vi "Initialize Attributes (public).vi"(8 "error in (no error)":errorcluster, 10 "Attribute Data":variant, 11 "CS++Base in":refnum<class "CS++Base.lvclass">) -> (0 "error out":errorcluster, 2 "Found?":bool, 3 "CS++Base out":refnum<class "CS++Base.lvclass">)   [LabVIEW 2015, in "CS++BaseClasses.lvlib" / "CS++Base.lvclass"]
doc: "Initialize object attribute.\n\nUnique resources should be allocated elsewhere!"
uses:
  CS++Base.lvclass
  CS++Base.lvclass/CS++Base.ctl
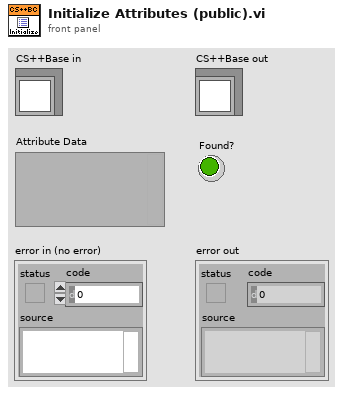
[diagram p1: front panel]
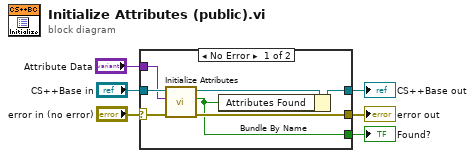
[diagram p0: block diagram]
diagram:
  n1 = case shown="No Error" "error in (no error)" {
    selector: "error in (no error)" -> [w12 w15]
    tunnel: [w11 w15] -> w5
    tunnel: [w8 w14] -> w3
    tunnel: "CS++Base in" -> [w13 w14]
    tunnel: "Attribute Data" -> [w10 _]
    tunnel: [w7 _] -> w1
    frame No Error {
      n2 = call-dynamic "Initialize Attributes.vi"("error in (no error)"=w12, "Attribute Data"=w10, "CS++Base in"=w13) -> ("error out"=w11:errorcluster, "Found?"=w7:bool, "CS++Base out"=w9:refnum<class "CS++Base.lvclass">)  [unwired: 6 in]
      n3 = Bundle By Name(cluster=w9, "Attributes Found"=w7) -> (w8:refnum<class "CS++Base.lvclass">)
    }
    frame Error {
    }
  }
  "error out" <- w5
  "CS++Base out" <- w3
  "Found?" <- w1
